vi "Check Limits.vi"(7 "Target":T2={"Position"=1.0, "Invert"=FALSE} {"Position" min=-0.5 max=0.5 step=0.1 format="%.2g"}, 8 "States":T1 format="%.4f") -> (0 "Off Track":bool, 1 "In Range":bool, 2 "Done":bool, 3 "In Range Seconds":dbl)   [LabVIEW 2018]
uses:
  Target.ctl
  States.ctl
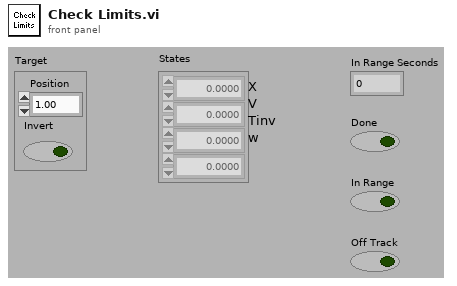
[diagram p1: front panel]
types:
  T1 = typedef "States.ctl" = dbl[]
  T2 = typedef "Target.ctl" = cluster{"Position":dbl, "Invert":bool}
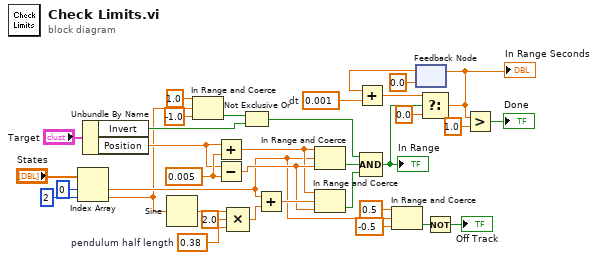
[diagram p0: block diagram]
diagram:
  w8 = 0.38  # pendulum half length
  w9 = 0.001  # dt
  w13 = 0.005 ("y")
  n1 = Index Array(array="States", index #1=0 ("index"), index #2=2 ("index")) -> (element #1=w4:dbl, element #2=w3:dbl)
  n2 = Unbundle By Name("Target") -> ("Invert"=w26:bool, "Position"=w12:dbl)
  n3 = Sine(x=w3) -> (sin(x)=w17:dbl)
  n4 = In Range and Coerce(upper limit=1.0, x=w3, lower limit=-1.0) -> (In Range?=w25:bool)  [unwired: 1 out]
  n5 = Add(x=w12, y=w13) -> (x+y=w19:dbl)
  n6 = Subtract(x=w12, y=w13) -> (x-y=w22:dbl)
  n7 = Compound Arithmetic op=MULTIPLY(w17, 2.0 ("value"), w8) -> (w18:dbl)
  n8 = Not Exclusive Or(1:w26, 2:w25) -> (0:w27:bool)
  n9 = Add(x=w4, y=w18) -> (x+y=w31:dbl)
  n10 = In Range and Coerce(upper limit=w19, x=w4, lower limit=w22) -> (In Range?=w28:bool)  [unwired: 1 out]
  n11 = In Range and Coerce(upper limit=w19, x=w31, lower limit=w22) -> (In Range?=w29:bool)  [unwired: 1 out]
  n12 = Compound Arithmetic op=AND(w27, w28, w29) -> (w30:bool)
  "In Range" <- w30
  n13 = In Range and Coerce(upper limit=0.5, x=w4, lower limit=-0.5) -> (In Range?=w34:bool)  [unwired: 1 out]
  n14 = feedback #1(0.0 ("f")) -> (w14:dbl)
  n15 = Add(x=w14, y=w9) -> (x+y=w15:dbl)
  n16 = Select(t=w15, s=w30, f=0.0) -> (s? t:f=w1:dbl)
  "In Range Seconds" <- w1
  n17 = feedback-in #1(w1) -> ()
  n18 = Not(x=w34) -> (.not. x?=→"Off Track":bool)
  n19 = Greater?(x=w1, y=1.0) -> (0:→"Done":bool)
